vi "parse_simulator_config.vi"(4 "error in":errorcluster, 6 "Simulator Configuration":string, 7 "simx in":T1) -> (0 "error out":errorcluster, 3 "simx out":T1)   [LabVIEW 2025]
uses:
  controls/simx_connection.ctl
  controls/config.ctl
  controls/trajectory.ctl
  controls/weather.ctl
  controls/connections.ctl
  controls/start_points.ctl
  <vilib>/Utility/miscctls.llb/LVBoundsTypeDef.ctl
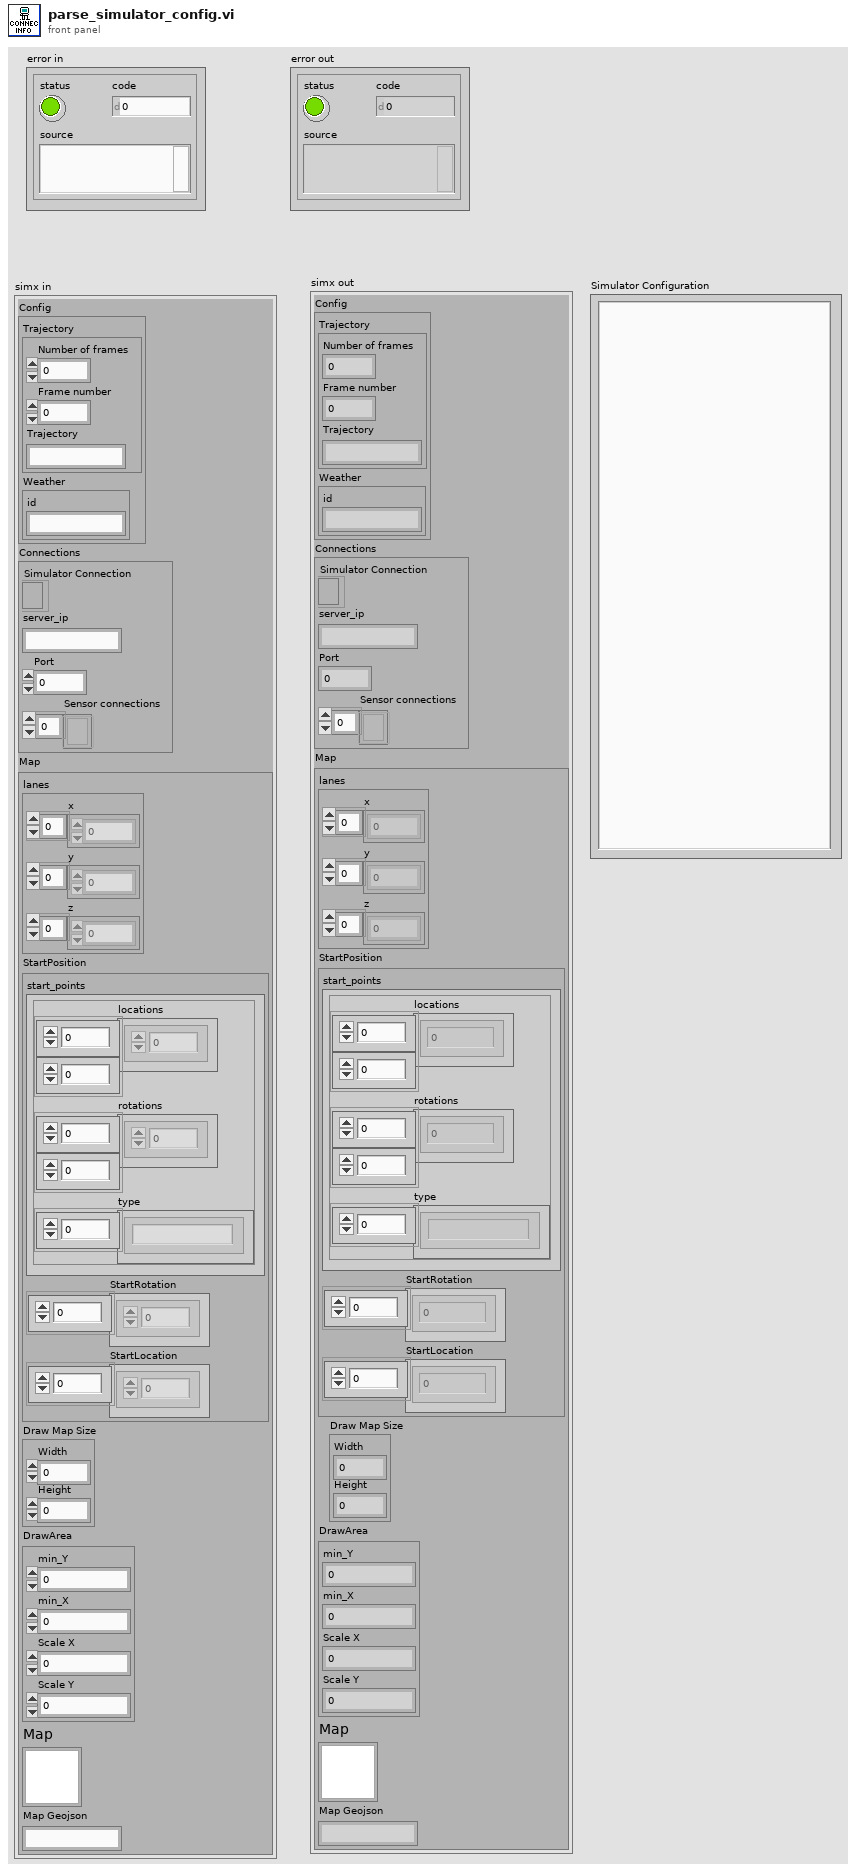
[diagram p1: front panel]
types:
  T1 = typedef "simx_connection.ctl" = cluster{"Config":T2, "Connections":T5, "Map":cluster{"lanes":cluster{"x":dbl[], "y":dbl[], "z":dbl[]}, "StartPosition":cluster{"start_points":T6, "StartRotation":dbl[], "StartLocation":dbl[]}, "Draw Map Size":T7, "DrawArea":cluster{"min_Y":dbl, "min_X":dbl, "Scale X":dbl, "Scale Y":dbl}, "Map":picture, "Map Geojson":string}}
  T2 = typedef "config.ctl" = cluster{"Trajectory":T3, "Weather":T4}
  T3 = typedef "trajectory.ctl" = cluster{"Number of frames":i32, "Frame number":i32, "Trajectory":string}
  T4 = typedef "weather.ctl" = cluster{"id":string}
  T5 = typedef "connections.ctl" = cluster{"Simulator Connection":refnum<k5>, "server_ip":string, "Port":i32, "Sensor connections":refnum<k5>[]}
  T6 = typedef "start_points.ctl" = cluster{"locations":dbl[][], "rotations":dbl[][], "type":string[]}
  T7 = typedef "LVBoundsTypeDef.ctl" = cluster{"Width":u32, "Height":u32}
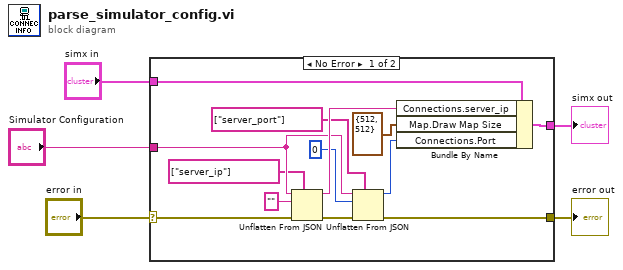
[diagram p0: block diagram]
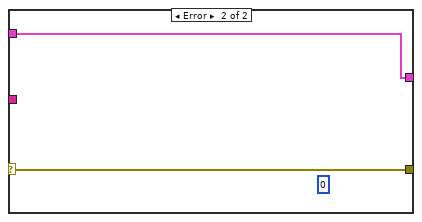
[diagram p2: hidden frame]
diagram:
  n1 = case shown="No Error" "error in" {
    selector: "error in" -> [w7 w20]
    tunnel: "simx in" -> [w18 w19]
    tunnel: [w16 w20] -> w4
    tunnel: "Simulator Configuration" -> [w14 _]
    tunnel: [w9 w19] -> w2
    frame No Error {
      n2 = Unflatten From JSON(path=string[] ["server_ip"], JSON string=w14, type and defaults="" ("regular expression"), error in (no error)=w7) -> (value=w17:string, error out=w15:errorcluster)  [unwired: 3 in]
      n3 = Unflatten From JSON(path=string[] ["server_port"], JSON string=w14, type and defaults=0 ("regular expression"), error in (no error)=w15) -> (value=w6:i32, error out=w16:errorcluster)  [unwired: 3 in]
      n4 = Bundle By Name(cluster=w18, "Connections.server_ip"=w17, "Map.Draw Map Size"=T7 {"Width"=512, "Height"=512}, "Connections.Port"=w6) -> (w9:T1)
    }
    frame Error {
      (unwired) 0 ("regular expression")
    }
  }
  "error out" <- w4
  "simx out" <- w2
